vi "Open Form.vi"(8 "error in (no error)":errorcluster, 10 "Form path":path, 11 "Form Model in":refnum<class "Form Model.lvclass">) -> (0 "error out":errorcluster, 3 "Form Model out":refnum<class "Form Model.lvclass">)   [LabVIEW 2020, in "Form Model.lvlib" / "Form Model.lvclass"]
uses:
  Form Model.lvclass
  C:/Program Files (x86)/National Instruments/LabVIEW 2020/vi.lib/ActorFramework/Actor/Actor.lvclass
  <vilib>/ActorFramework/Actor/Actor.lvclass/Actor.ctl
  Form Model.lvclass/Form Model.ctl
  Form Configuration/Form Model Configuration.lvclass/Form Model Configuration.ctl
  Form Server Messages Messages/Open Form Msg/Open Form Msg.lvclass/Open Form Msg.ctl
  <vilib>/ActorFramework/Message Enqueuer/Message Enqueuer.lvclass/Message Enqueuer.ctl
  <vilib>/ActorFramework/Message Enqueuer/Enqueue.vi
  Form Server Messages Messages/Open Form Msg/Open Form Msg.lvclass
  C:/Program Files (x86)/National Instruments/LabVIEW 2020/vi.lib/ActorFramework/Message/Message.lvclass
  <vilib>/ActorFramework/Message Priority Queue/Priority Enqueue.vi
  Form Configuration/Form Model Configuration.lvclass
  <vilib>/ActorFramework/Actor/Actor.lvclass
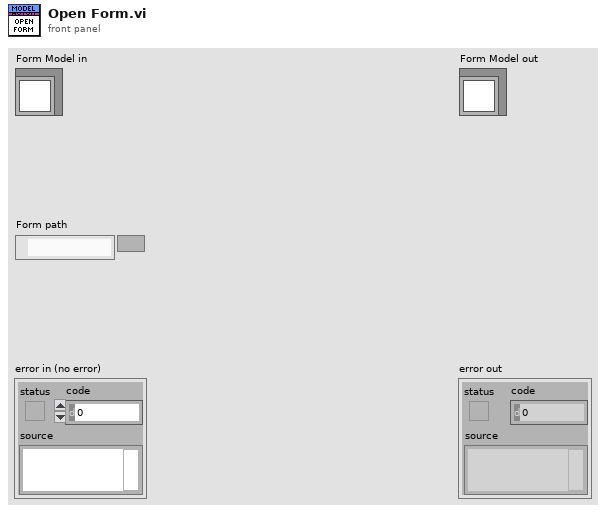
[diagram p1: front panel]
types:
  T1 = typedef "Form Server Interfaces.lvlib/Form ID.ctl" = cluster{"Name":string, "Panel type":string}
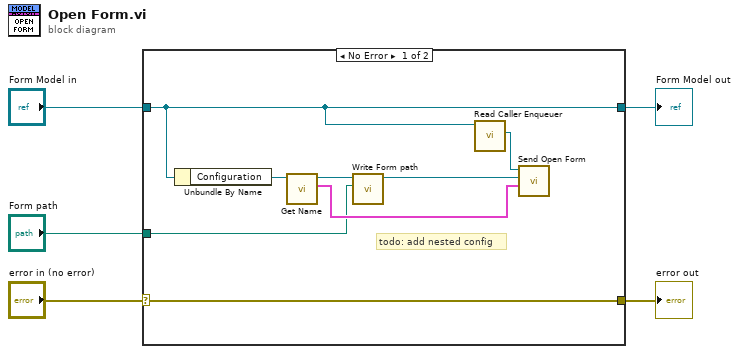
[diagram p0: block diagram]
diagram:
  n1 = case shown="No Error" "error in (no error)" {
    selector: "error in (no error)" -> [w13 w15]
    tunnel: "Form Model in" -> [w11 w14]
    tunnel: [w13 w15] -> w3
    tunnel: [w11 w14] -> w2
    tunnel: "Form path" -> [w7 _]
    frame No Error {
      # "todo: add nested config"
      n2 = Unbundle By Name(w11) -> ("Configuration"=w12:refnum<class "Form Model Configuration.lvclass">)
      n3 = call-dynamic "Get Name.vi"("Form Configuration in"=w12) -> ("Form ID"=w9:T1, "Form Configuration out"=w8:refnum<class "Form Model Configuration.lvclass">)  [unwired: 8 in, 1 out]
      n4 = call "Write Form path.vi"("Form path"=w7, "Form Configuration in"=w8) -> ("Form Configuration out"=w6:refnum<class "Form Model Configuration.lvclass">)  [unwired: 8 in, 1 out]
      n5 = call <vilib>:"Read Caller Enqueuer.vi"("Actor"=w11) -> ("Caller Enqueuer"=w10:refnum<class "Message Enqueuer.lvclass">)  [unwired: 10 in]
      n6 = call "Send Open Form.vi"("Caller Name"=w9, "Form Config"=w6, "Message Enqueuer"=w10) -> ()  [unwired: 7 in, 2 out]
    }
    frame Error {
    }
  }
  "error out" <- w3
  "Form Model out" <- w2
